vi "PC Main.vi"() -> ()   [LabVIEW 2021]
uses:
  Variable custer.ctl
panel:
  out "data out":u32(colorbox)
  in  "stop":bool
  in  "Color":u32(colorbox)
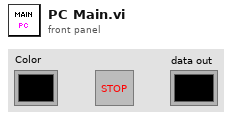
[diagram p1: front panel]
types:
  T1 = typedef "Variable custer.ctl" = cluster{"Prefix":string, "IP":string, "Librery name":string, "Variable name":string}
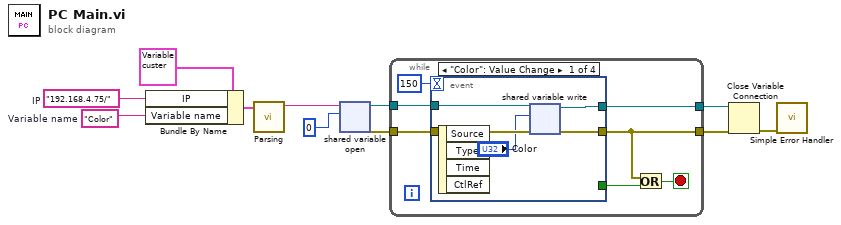
[diagram p0: block diagram]
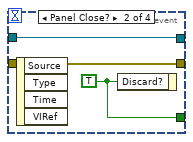
[diagram p2: hidden frame]
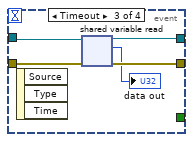
[diagram p3: hidden frame]
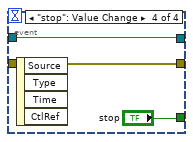
[diagram p4: hidden frame]
diagram:
  w3 = "Color"  # Variable name
  w4 = "192.168.4.75/"  # IP
  n1 = Bundle By Name(cluster=T1 {"Prefix"="ni.var.psp://", "IP"="", "Librery name"="Shared Variable/", "Variable name"=""}, "IP"=w4, "Variable name"=w3) -> (w2:T1)
  n2 = call "Parsing.vi"("Cluster"=w2) -> ("String"=w1:string)  [unwired: 4 in]
  n3 = shared-variable-open(w1, u32 0) -> (w7:refnum<k21>, w10:errorcluster)  [unwired: 2 in]
  n4 = while {
    tunnel: w7 -> [w18]
    tunnel: [w17] -> w8
    tunnel: [w15] -> w9
    tunnel: w10 -> [w16]
    stop <- w14 stop-if-true
    n5 = event shown="[0] \"Color\": Value Change" {
      selector: _ -> [_ _ _ _]
      dyn-events: _ -> [_ _ _ _]
      timeout: 150 -> [_ _ _ _]
      tunnel: w18 -> [w23 w25 w29 w32]
      tunnel: [w22 w25 w30 w32] -> w17
      tunnel: w16 -> [w21 w24 w28 w33]
      tunnel: [w20 w24 w31 w33] -> w15
      tunnel: [_ w26 _ "stop"] -> w13
      event "Color": Value Change {
        n6 = event-data() -> ()  [unwired: 1 in, 4 out]
        n7 = shared-variable-write(w23, w21, "Color") -> (w22:refnum<k21>, w20:errorcluster)
      }
      event Panel Close? {
        w26 = TRUE
        n8 = event-data() -> ()  [unwired: 1 in, 4 out]
        n9 = event-data("Discard?"=w26) -> ()  [unwired: 1 in, 1 out]
      }
      event Timeout {
        n10 = event-data() -> ()  [unwired: 1 in, 3 out]
        n11 = shared-variable-read(w29, w28) -> (w30:refnum<k21>, w31:errorcluster, →"data out":u32)  [unwired: 1 out]
      }
      event "stop": Value Change {
        n12 = event-data() -> ()  [unwired: 1 in, 4 out]
      }
    }
    n13 = Or(x=w15, y=w13) -> (x .or. y?=w14:bool)
  }
  n14 = Close Variable Connection(8:w9, 11:w8) -> (0:w11:errorcluster)
  n15 = call <vilib>:"Simple Error Handler.vi"("error in (no error)"=w11) -> ()  [unwired: 4 in, 5 out]
